vi "SEGUIDOR_DE_PAREDE.vi"(2 "NXT/EV3":T1) -> (0 "NXT/EV3 2":T1)   [LabVIEW 2016]
uses:
  <vilib>/NXT/Subs/LVHSConnector.ctl
  <vilib>/NXT/LegoClasses/BrickReference/BrickReference.lvclass
  <vilib>/NXT/Block Support/NXT_OutputPort.ctl
  <vilib>/NXT/Block Support/NXT_InputPort.ctl
  <vilib>/NXT/NXTIO Xnodes/NXTIONodeSubVIs/NXTMoveMotors.vi
  <vilib>/NXT/Dual Mode Library/Sensors/EV3_Ultrasonic_CM.vi
  <vilib>/NXT/Dual Mode Library/Sensors/Touch_Pressed.vi
  <vilib>/NXT/NXTIO Xnodes/AddressXNode/NXTIOAddress.xnode
  <vilib>/NXT/NXTIO Xnodes/NXTIOXNode/NXTIO.xnode
panel:
  in  "Kp":sgl
  in  "Dmin":sgl
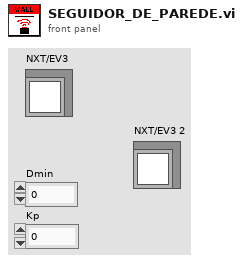
[diagram p1: front panel]
types:
  T1 = typedef "LVHSConnector.ctl" = refnum<class "BrickReference.lvclass">
  T2 = typedef "NXT_OutputPort.ctl" = u8
  T3 = typedef "NXT_InputPort.ctl" = u32
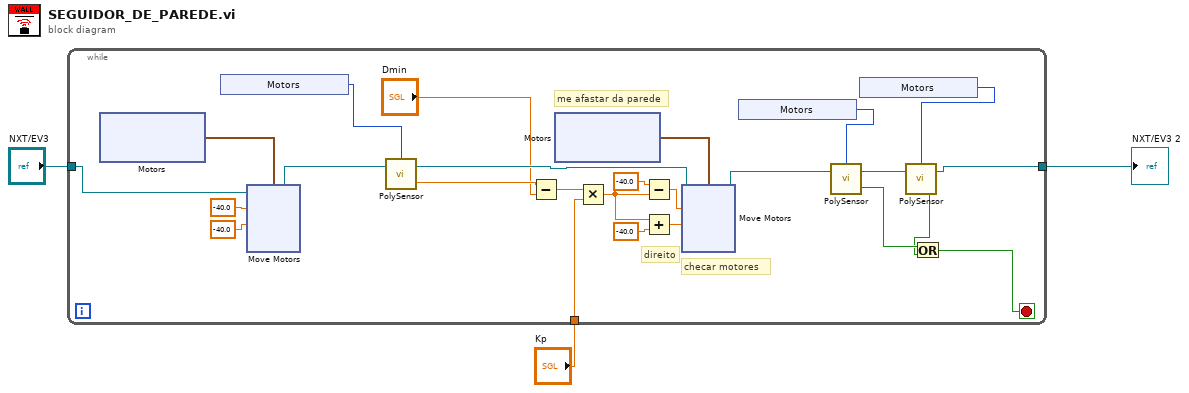
[diagram p0: block diagram]
diagram:
  n1 = while {
    tunnel: "NXT/EV3" -> [w25]
    tunnel: [w13] -> w2
    tunnel: "Kp" -> [w22]
    stop <- w10 stop-if-true
    # "direito"
    # "me afastar da parede"
    # "checar motores"
    n2 = xnode "Motors"() -> ("Motor"=w27:cluster{"Port":T2, "Port":T2})
    n3 = xnode "Motors"() -> ("Sensor"=w9:T3)
    n4 = xnode "Move Motors"("Power/Speed 2"=sgl -40.0 ("x"), "Power/Speed 1"=sgl -40.0 ("x"), "Motors"=w27, "NXT/EV3"=w25) -> ("NXT/EV3"=w26:T1)
    n5 = call-poly <vilib>:"PolySensor.vi"("NXT/EV3"=w26, "Port (Port 1)"=w9) -> ("Centimeters"=w5:sgl, "NXT/EV3"=w28:T1)  [unwired: 1 in]
    n6 = Subtract(x=w5, y="Dmin") -> (x-y=w18:sgl)
    n7 = xnode "Motors"() -> ("Motor"=w19:cluster{"Port":T2, "Port":T2})
    n8 = Multiply(x=w18, y=w22) -> (x*y=w20:sgl)
    n9 = Subtract(x=sgl -40.0, y=w20) -> (x-y=w16:sgl)
    n10 = Add(x=w20, y=sgl -40.0 ("x")) -> (x+y=w17:sgl)
    n11 = xnode "Move Motors"("Power/Speed 2"=w17, "Power/Speed 1"=w16, "Motors"=w19, "NXT/EV3"=w28) -> ("NXT/EV3"=w14:T1)
    n12 = xnode "Motors"() -> ("Sensor"=w8:T3)
    n13 = call-poly <vilib>:"PolySensor.vi"("NXT/EV3"=w14, "Port (Port 1)"=w8) -> ("Yes / No"=w12:bool, "NXT/EV3"=w15:T1)  [unwired: 1 in]
    n14 = xnode "Motors"() -> ("Sensor"=w7:T3)
    n15 = call-poly <vilib>:"PolySensor.vi"("NXT/EV3"=w15, "Port (Port 1)"=w7) -> ("Yes / No"=w11:bool, "NXT/EV3"=w13:T1)  [unwired: 1 in]
    n16 = Or(x=w12, y=w11) -> (x .or. y?=w10:bool)
  }
  "NXT/EV3 2" <- w2
